vi "iRobot Example - Square.vi"() -> ()   [LabVIEW 2013]
doc: "Drives the iRobot in a square using a single loop to poll distance and angle traveled."
uses:
  Advanced/UART/iRobot UART Port Type.ctl
  Actuator/Drive Direction.ctl
panel:
  in  "UART port in":T1="ASRL1::INSTR"
  in  "stop":bool
  in  "Max Wheel Speed (mm/s)":i16=250
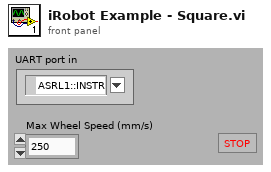
[diagram p1: front panel]
types:
  T1 = typedef "iRobot UART Port Type.ctl" = refnum<visa-resource-name>
  T2 = typedef "Drive Direction.ctl" = u16
  T3 = typedef "Sensor Group 6.ctl" = cluster{"Bumps + Wheel Drops":T4, "Wall":bool, "Cliff Left":bool, "Cliff Front Left":bool, "Cliff Front Right":bool, "Cliff Right":bool, "Virtual Wall":bool, "Low-Side Driver + Wheel Overcurrent":T5, "Infrared":u8, "Buttons":T6, "Distance (mm)":i32, "Angle (deg)":i32, "Charging State":T7, "Voltage (mV)":u16, "Current (mA)":i16, "Battery Temperature (deg C)":i8, "Battery Charge (mAh)":u16, "Battery Capacity (mAh)":u16, "Wall Signal (0-4095)":u16, "Cliff Left Signal (0-4095)":u16, "Cliff Front Left Signal (0-4095)":u16, "Cliff Front Right Signal (0-4095)":u16, "Cliff Right Signal (0-4095)":u16, "Cargo Bay Digital Inputs":T8, "Cargo Bay Analog Signal (0-1023)":u16, "Charging Sources Available":T9, "OI Mode":T10, "Song Number":u8, "Song Playing":bool, "Number of Stream Packets":u8, "Requested Velocity (mm/s)":i16, "Requested Radius (mm)":i16, "Requested Right Wheel Velocity (mm/s)":i16, "Requested Left Wheel Velocity (mm/s)":i16}
  T4 = typedef "Bumps + Wheel Drops.ctl" = cluster{"Wheeldrop Caster":bool, "Wheeldrop Left":bool, "Wheeldrop Right":bool, "Bump Left":bool, "Bump Right":bool}
  T5 = typedef "Low-Side Driver + Wheel Overcurrent.ctl" = cluster{"Low-Side Driver 0":bool, "Low-Side Driver 1":bool, "Low-Side Driver 2":bool, "Left Wheel":bool, "Right Wheel":bool}
  T6 = typedef "Buttons.ctl" = cluster{"Advance":bool, "Play":bool}
  T7 = typedef "Charging State.ctl" = enum16{"Not Charging", "Reconditioning Charging", "Full Charging", "Trickle Charging", "Waiting", "Charging Fault Condition"}
  T8 = typedef "Cargo Bay Digital Inputs.ctl" = cluster{"Digital Input 0":bool, "Digital Input 1":bool, "Digital Input 2":bool, "Digital Input 3":bool, "Device Detect":bool}
  T9 = typedef "Charging Sources Available.ctl" = cluster{"Internal Charger":bool, "Home Base":bool}
  T10 = typedef "OI Mode.ctl" = enum16{"Off", "Passive", "Safe", "Full"}
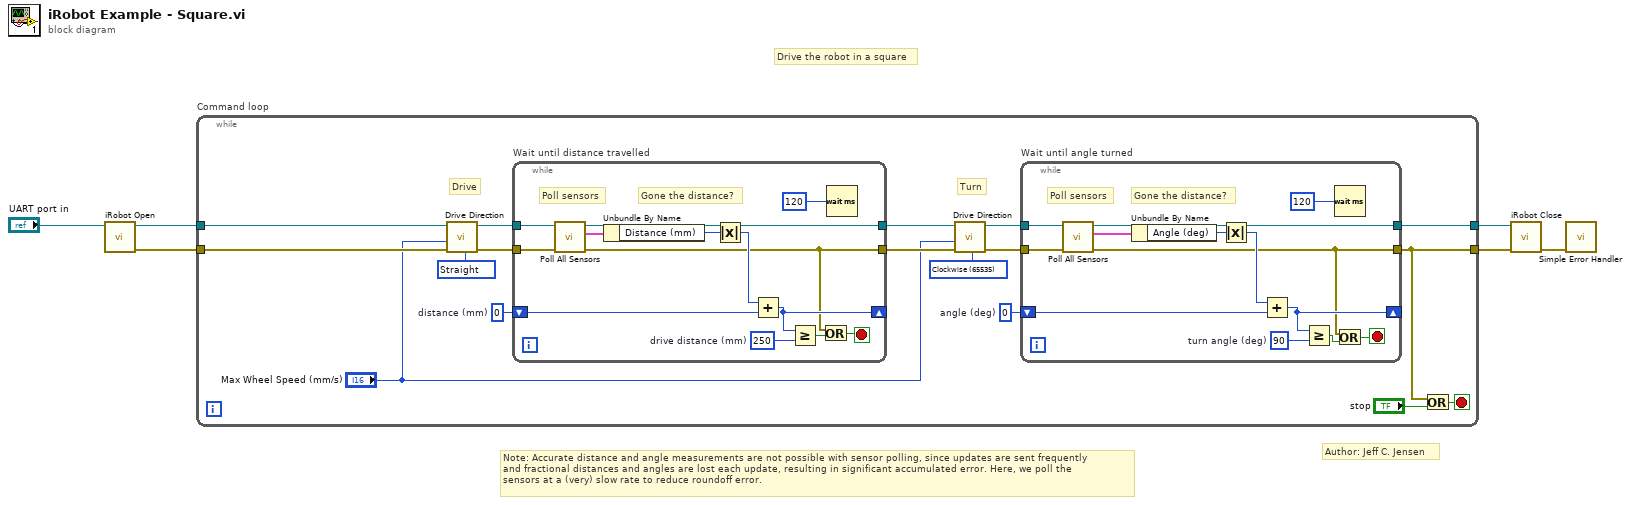
[diagram p0: block diagram]
diagram:
  # "Author: Jeff C. Jensen"
  # "Drive the robot in a square"
  # "Note: Accurate distance and angle measurements are not possible with sensor polling, since updates are sent frequently\nand fractional distances and angles are lost each update, resulting in significant accumulated error. Here, we poll the\nsensors at a (very) slow rate to reduce roundoff error."
  n1 = call "iRobot Open.vi"("UART port in"="UART port in") -> ("error out"=w5:errorcluster, "UART port out"=w6:T1)  [unwired: 9 in]
  n2 = while "Command loop" {
    tunnel: w6 -> [w15]
    tunnel: w5 -> [w14]
    tunnel: [w9] -> w3
    tunnel: [w11] -> w4
    stop <- w10 stop-if-true
    w18 = T2 32768 items=["Straight"=32768, "Clockwise"=65535, "Counter-Clockwise"=1] ("iRobot Drive Direction")
    w17 = 0  # distance (mm)
    w21 = T2 65535 items=["Straight"=32768, "Clockwise"=65535, "Counter-Clockwise"=1] ("iRobot Drive Direction")
    w22 = 0  # angle (deg)
    # "Drive"
    # "Turn"
    n3 = call "Drive Direction.vi"("error in"=w14, "Velocity (mm/s)"="Max Wheel Speed (mm/s)", "iRobot Drive Direction"=w18, "UART port in"=w15) -> ("error out"=w19:errorcluster, "UART port out"=w16:T1)  [unwired: 6 in]
    n4 = while "Wait until distance travelled" {
      tunnel: w16 -> [w31]
      shift-right: [w33] -> _
      shift-left: w17 -> [w34]
      tunnel: w19 -> [w28]
      tunnel: [w24] -> w13
      tunnel: [w27] -> w12
      stop <- w25 stop-if-true
      w36 = 250  # drive distance (mm)
      # "Gone the distance?"
      # "Poll sensors"
      n5 = call "Poll All Sensors.vi"("error in"=w28, "UART port in"=w31) -> ("error out"=w24:errorcluster, "iRobot Sensors"=w30:T3, "UART port out"=w27:T1)  [unwired: 6 in, 1 out]
      n6 = Unbundle By Name(w30) -> ("Distance (mm)"=w35:i32)
      n7 = Absolute Value(x=w35) -> (abs(x)=w32:i32)
      n8 = Add(x=w32, y=w34) -> (x+y=w33:i32)
      n9 = Greater Or Equal?(x=w33, y=w36) -> (x >= y?=w26:bool)
      n10 = Or(x=w24, y=w26) -> (x .or. y?=w25:bool)
      n11 = Wait (ms)(milliseconds to wait=u32 120) -> ()  [unwired: 1 out]
    }
    n12 = call "Drive Direction.vi"("error in"=w13, "Velocity (mm/s)"="Max Wheel Speed (mm/s)", "iRobot Drive Direction"=w21, "UART port in"=w12) -> ("error out"=w20:errorcluster, "UART port out"=w23:T1)  [unwired: 6 in]
    n13 = while "Wait until angle turned" {
      tunnel: w23 -> [w44]
      shift-right: [w46] -> _
      shift-left: w22 -> [w47]
      tunnel: w20 -> [w41]
      tunnel: [w38] -> w9
      tunnel: [w37] -> w11
      stop <- w39 stop-if-true
      w49 = 90  # turn angle (deg)
      # "Gone the distance?"
      # "Poll sensors"
      n14 = call "Poll All Sensors.vi"("error in"=w41, "UART port in"=w44) -> ("error out"=w38:errorcluster, "iRobot Sensors"=w43:T3, "UART port out"=w37:T1)  [unwired: 6 in, 1 out]
      n15 = Unbundle By Name(w43) -> ("Angle (deg)"=w48:i32)
      n16 = Absolute Value(x=w48) -> (abs(x)=w45:i32)
      n17 = Add(x=w45, y=w47) -> (x+y=w46:i32)
      n18 = Greater Or Equal?(x=w46, y=w49) -> (x >= y?=w40:bool)
      n19 = Wait (ms)(milliseconds to wait=u32 120) -> ()  [unwired: 1 out]
      n20 = Or(x=w38, y=w40) -> (x .or. y?=w39:bool)
    }
    n21 = Or(x=w9, y="stop") -> (x .or. y?=w10:bool)
  }
  n22 = call "iRobot Close.vi"("error in"=w3, "UART port in"=w4) -> ("error out"=w2:errorcluster)  [unwired: 9 in]
  n23 = call <vilib>:"Simple Error Handler.vi"("error in (no error)"=w2) -> ()  [unwired: 4 in, 5 out]
